vi "init.vi"(8 "error in (no error)":errorcluster, 11 "USB IO in":refnum<class "USB IO.lvclass">) -> (0 "error out":errorcluster, 3 "USB IO out":refnum<class "USB IO.lvclass">)   [LabVIEW 2025, in "USB IO.lvlib" / "USB IO.lvclass"]
uses:
  USB IO.lvclass
  USB IO.lvclass/USB IO.ctl
  <vilib>/DAQmx/write.llb/DAQmx Write (Digital 1D Bool NChan 1Samp 1Line).vi
  <vilib>/DAQmx/create/channels.llb/DAQmx Create Channel (DO-Digital Output).vi
  <vilib>/DAQmx/miscellaneous.llb/DAQmx Fill In Error Info.vi
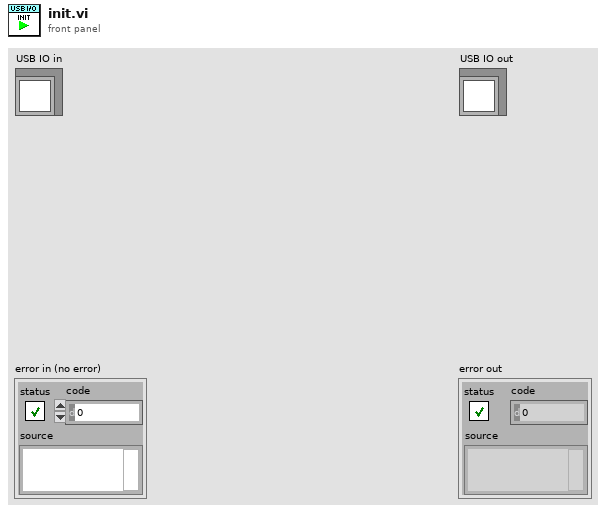
[diagram p1: front panel]
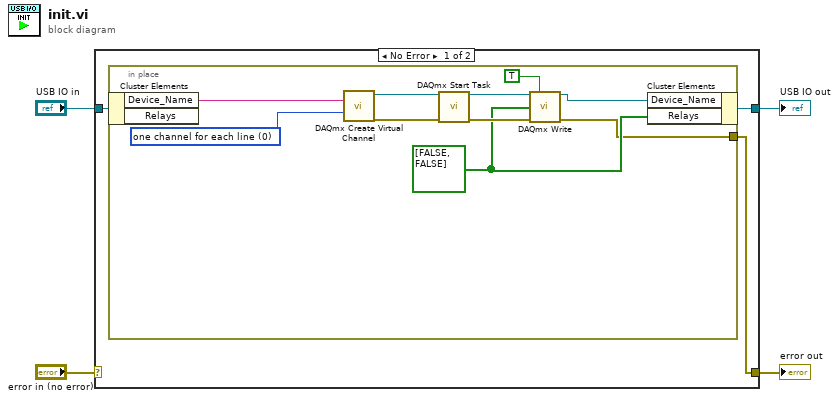
[diagram p0: block diagram]
diagram:
  n1 = case shown="No Error" "error in (no error)" {
    selector: "error in (no error)" -> [_ w19]
    tunnel: [w5 w19] -> w3
    tunnel: [w6 w18] -> w1
    tunnel: "USB IO in" -> [w7 w18]
    frame No Error {
      n2 = in-place {
        in-place-border: [w8] -> w5
        w9 = bool[] [FALSE, FALSE] ("data")
        w16 = 0 items=["one channel for each line", "one channel for all lines"] ("line grouping")
        n3 = in-place-cluster #1(w7) -> ("Device_Name"=w17:string)  [unwired: 1 out]
        n4 = call-poly <vilib>:"DAQmx Create Virtual Channel.vi"("lines"=w17, "line grouping"=w16) -> ("task out"=w15:refnum<k21>, "error out"=w14:errorcluster)  [unwired: 12 in]
        n5 = call <vilib>:"DAQmx Start Task.vi"("task/channels in"=w15, "error in"=w14) -> ("task out"=w13:refnum<k21>, "error out"=w12:errorcluster)  [unwired: 12 in]
        n6 = call-poly <vilib>:"DAQmx Write.vi"("task/channels in"=w13, "auto start"=TRUE, "data"=w9, "error in"=w12) -> ("task out"=w10:refnum<k21>, "error out"=w8:errorcluster)  [unwired: 9 in, 1 out]
        n7 = in-place-cluster #1("Device_Name"=w10, "Relays"=w9) -> (w6:refnum<class "USB IO.lvclass">)
      }
    }
    frame Error {
    }
  }
  "error out" <- w3
  "USB IO out" <- w1
